vi "GageAvgSpec_orionkhw.vi"() -> ()   [LabVIEW 2016]
uses:
  <vilib>/express/express analysis/Spectral/Block/exnSpectralBlock spectral measurements power poly.vi
  <vilib>/express/express analysis/Spectral/Block/exnSpectralBlock spectral measurements power WFM.vi
  <vilib>/Utility/file.llb/Write To Spreadsheet File (DBL).vi
  <vilib>/express/express analysis/Spectral/XNode/ExpressSpectralMeasurementsBlockNode.xnode
panel:
  out "Spec(ch0)":cluster{"f0":dbl, "df":dbl, "magnitude":dbl[]}(graph)
  out "Spec(ch2)":cluster{"f0":dbl, "df":dbl, "magnitude":dbl[]}(graph)
  out "100 세트 저장완료":bool
  in  "데이터 저장 시작":bool
  out "루프 사이의 time interval":dbl
  out "Spec(ch3)":cluster{"f0":dbl, "df":dbl, "magnitude":dbl[]}(graph)
  in  "Trigger":T1={"Slope"=0, "Level"=0, "Source"=0, "External Range"=2000, "External Coupling"=0, "External"=FALSE, "Disable"=FALSE, "External Impedance"=1} {"External Impedance" items=["50 Ohm", "HiZ"]; "External Coupling" items=["DC", "AC"]; "External Range" min=2000 max=10000 step=8000; "Slope" items=["Rising", "Falling"]; "Level" min=-100 max=100; "Source" min=0 max=64 step=1}
  in  "Averages":u32=1 min=1 step=1
  in  "Averaging Method":bool
  in  "Channels":T2(array[cluster])=[{"Coupling"=0, "Differential Input"=FALSE, "Direct-to-ADC"=FALSE, "Range"=2000, "Impedance"=50, "Filter"=0}] {"Impedance" min=50 max=1000000 step=999950; "Coupling" items=["DC", "AC"]}
  in  "Acquisition":T3={"Sample Rate"=50000000.0, "Mode"=2, "Depth"=8192.0, "Segment Size"=8192.0, "Trigger Timeout"=1000000.0, "Trigger Holdoff"=0.0, "Trigger Delay"=0.0, "Clock mode"=enum."Internal"} {"Segment Size" min=256.0 step=128.0; "Trigger Holdoff" min=0.0 step=128.0; "Trigger Delay" min=0.0 step=128.0; "Depth" min=256.0 step=128.0; "Mode" items=["Single", "Dual", "Quad", "Octal"]}
  in  "Continuous":bool=TRUE
  out "Progress":string
  in  "stop":bool
  out "System Name":string
  out "Sample Bits":i32
  out "Trigger Count":i32
  out "Channel Count":i32
  out "Board Count":i32
  out "System Count":i32
  in  "Points":u32=4096
  in  "Start":i32
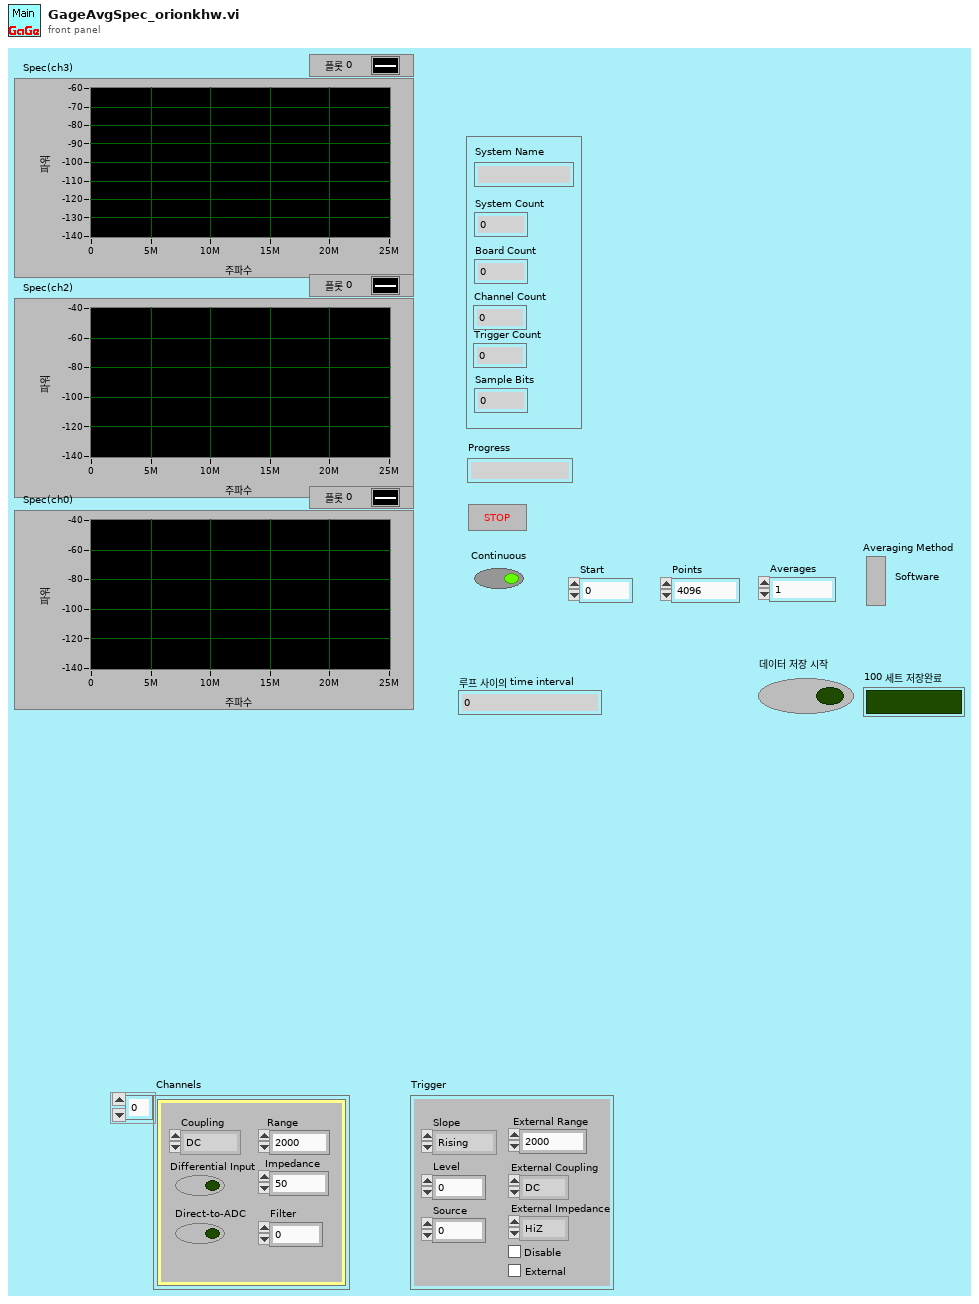
[diagram p1: front panel]
types:
  T1 = cluster{"Slope":u16, "Level":i32, "Source":i32, "External Range":u32, "External Coupling":u16, "External":bool, "Disable":bool, "External Impedance":u16}
  T2 = cluster{"Coupling":u16, "Differential Input":bool, "Direct-to-ADC":bool, "Range":u32, "Impedance":u32, "Filter":i32}[]
  T3 = cluster{"Sample Rate":dbl, "Mode":u16, "Depth":dbl, "Segment Size":dbl, "Trigger Timeout":dbl, "Trigger Holdoff":dbl, "Trigger Delay":dbl, "Clock mode":enum16{"Internal", "External", "Reference"}}
  T4 = cluster{"averaging mode":u16, "weighting mode":u16, "number of averages":u32}
  T5 = cluster{"dB On (F)":bool, "unwrap phase (F)":bool, "convert to degree (F)":bool}
  T6 = cluster{"Handle":u32, "Sample size":u32, "Resolution":i32, "Offset":i32, "Channels":u32, "Boards":u32}
  T7 = cluster{string, "Differential Input":bool, "Direct-to-ADC":bool, "Range":u32, "Impedance":u32, i32, "Filter":i32}
  T8 = cluster{"RingText.Text":string, "Level":i32, "Source":i32, "External Range":u32, "RingText.Text":string, "External":bool, "Disable":bool, "RingText.Text":string}
  T9 = cluster{"RingText.Text":string, "Level":i32, "Source":i32, "External Range":u32, "RingText.Text":string, "External":bool, "Disable":bool, "RingText.Text":string}[]
  T10 = cluster{"Handle":u32, "Sample Size":u32, "Resolution":i32, "Offset":i32, "Channels":u32, "Boards":u32}
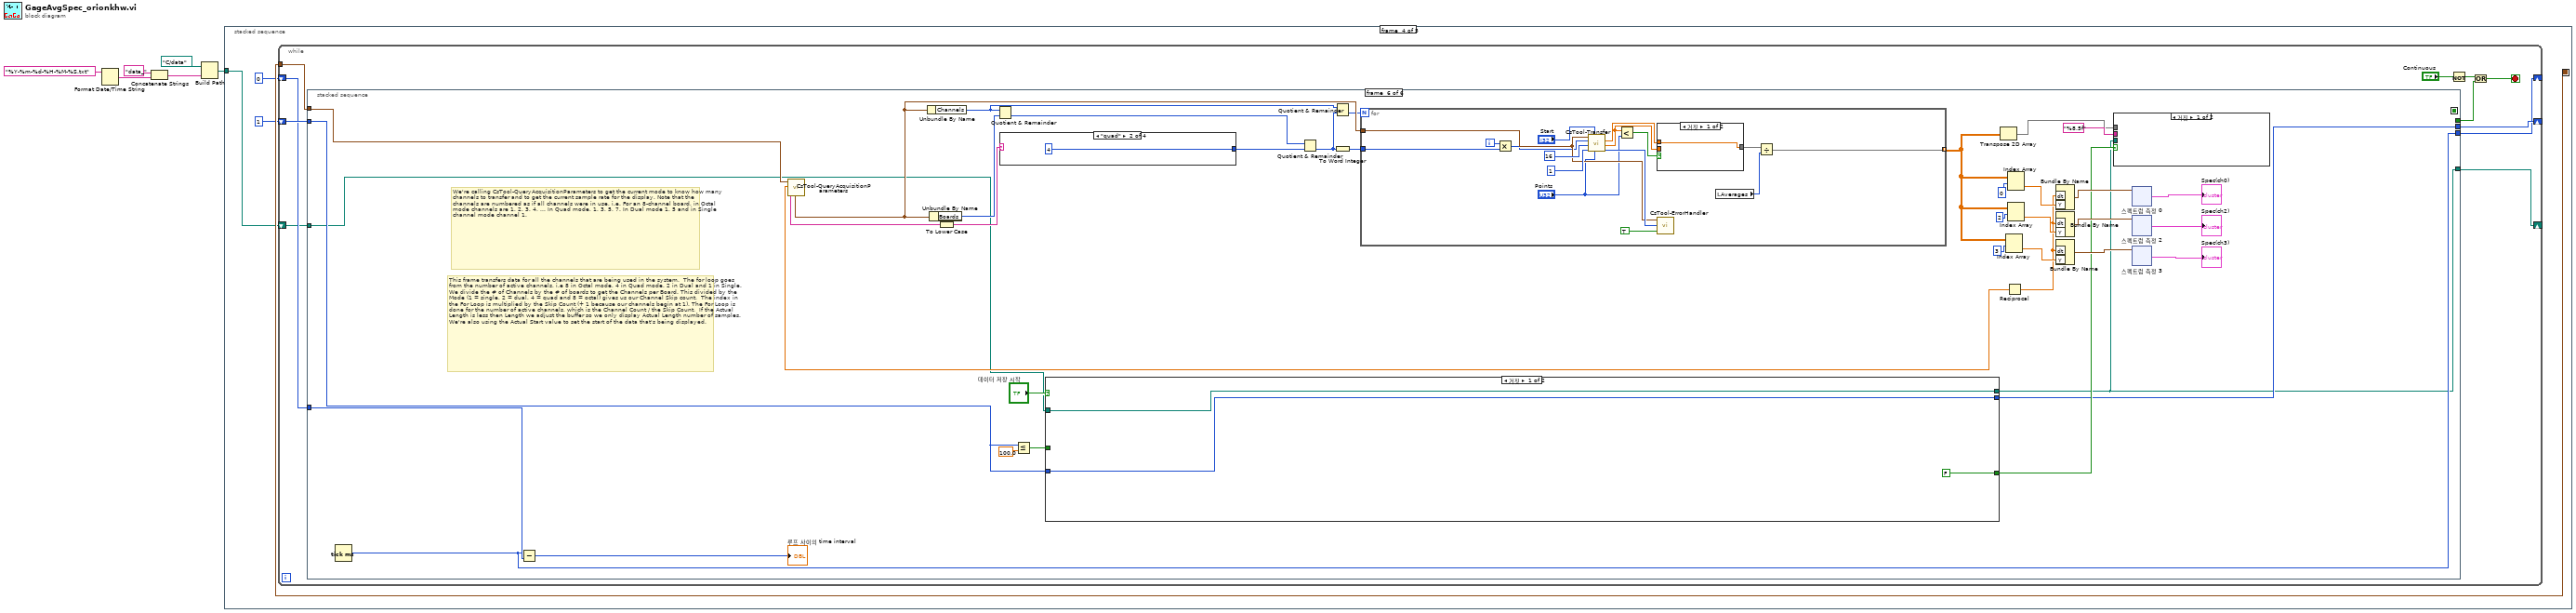
[diagram p0: block diagram]
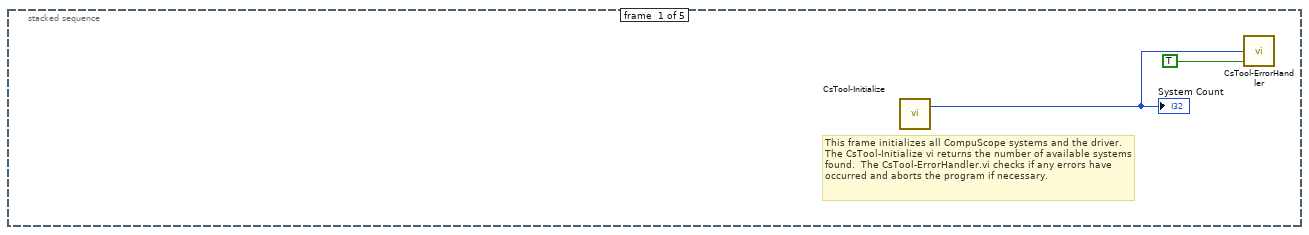
[diagram p2: hidden frame]
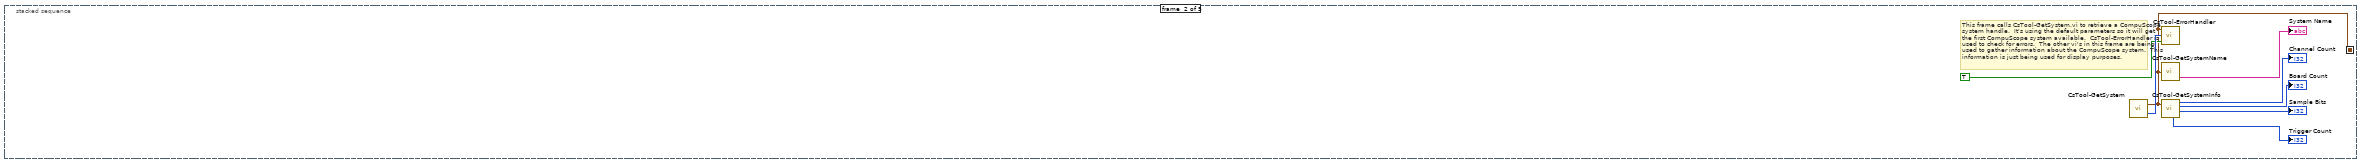
[diagram p3: hidden frame]
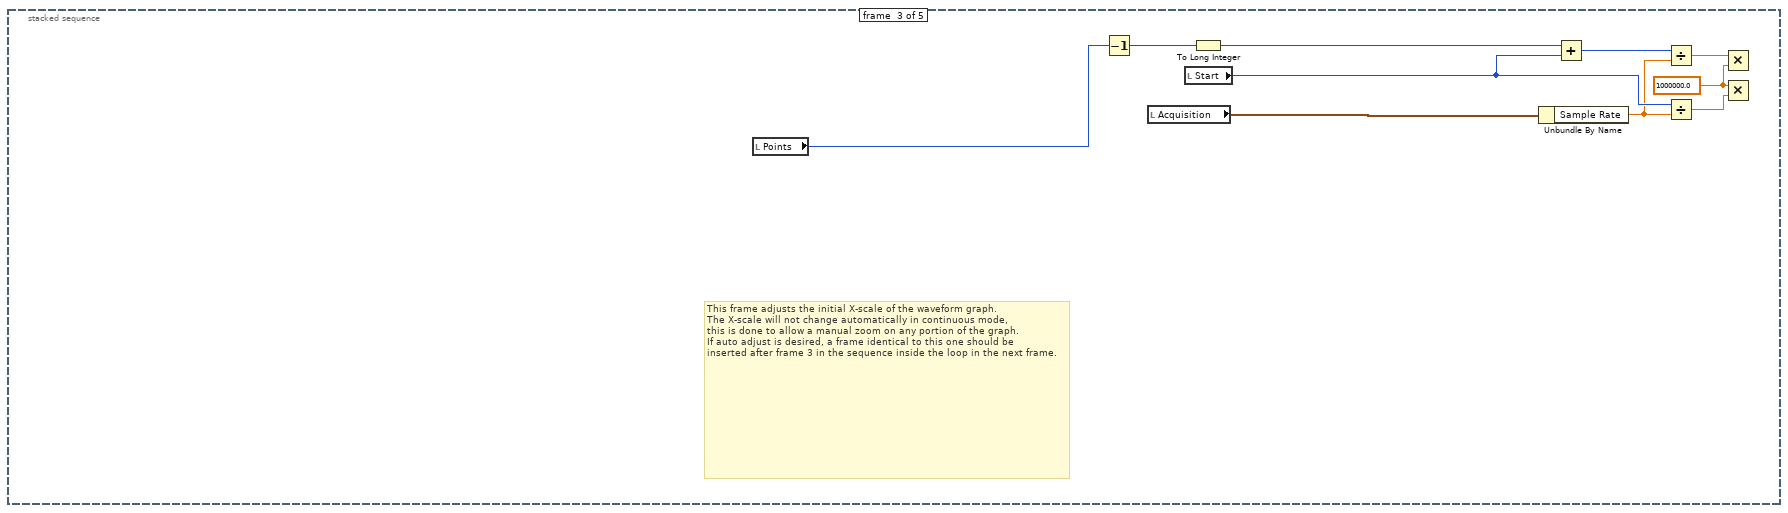
[diagram p4: hidden frame]
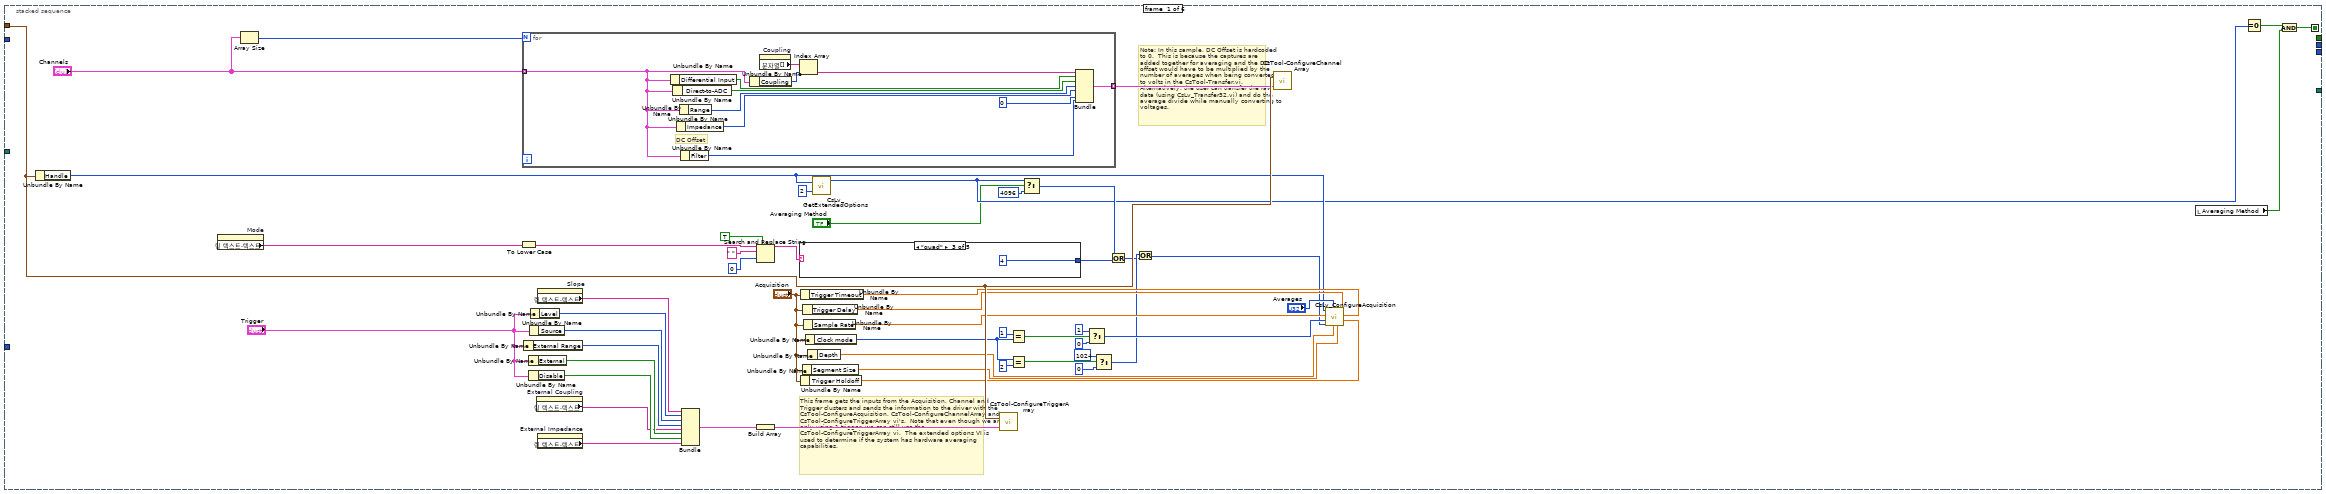
[diagram p5: hidden frame]
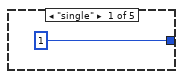
[diagram p6: hidden frame]
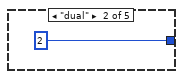
[diagram p7: hidden frame]
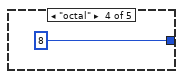
[diagram p8: hidden frame]
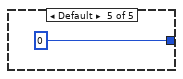
[diagram p9: hidden frame]
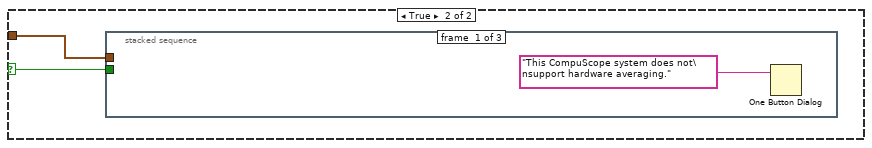
[diagram p11: hidden frame]
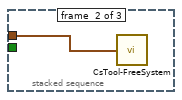
[diagram p12: hidden frame]
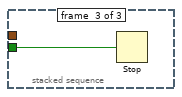
[diagram p13: hidden frame]
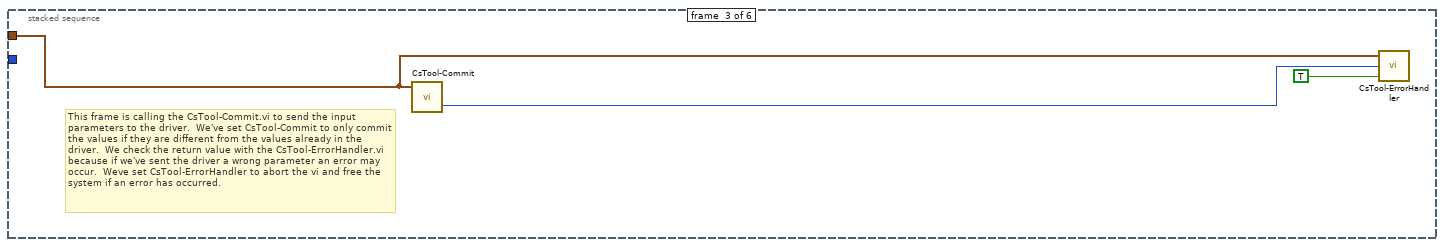
[diagram p14: hidden frame]
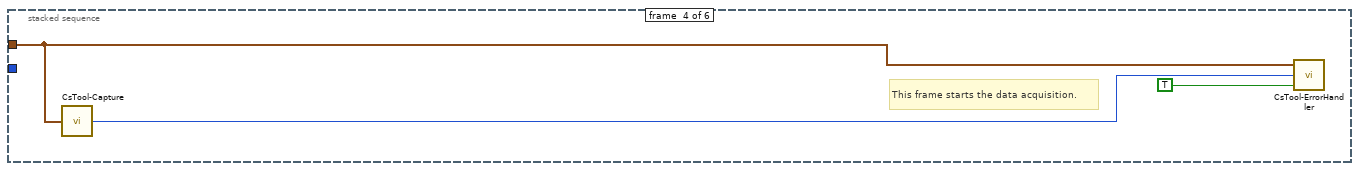
[diagram p15: hidden frame]
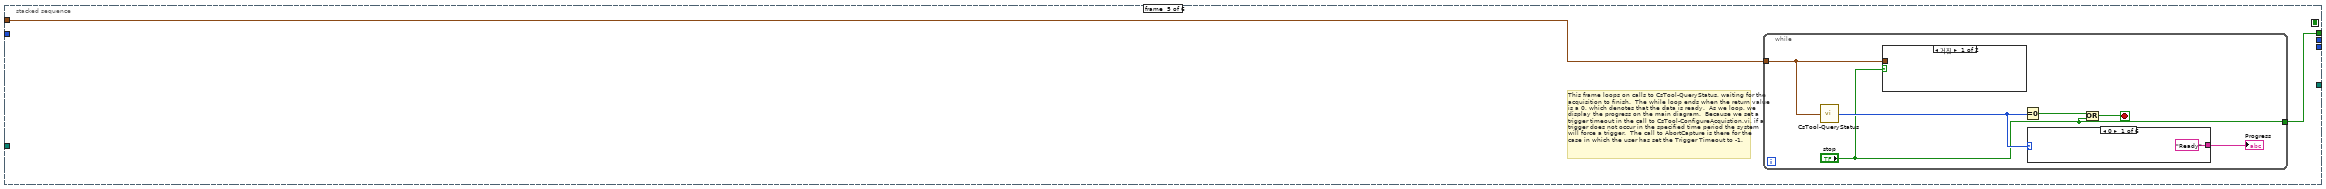
[diagram p16: hidden frame]
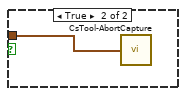
[diagram p17: hidden frame]
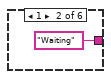
[diagram p18: hidden frame]
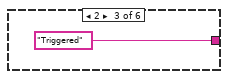
[diagram p19: hidden frame]
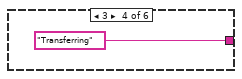
[diagram p20: hidden frame]
diagram:
  n1 = Format Date/Time String(time format string (%c)="%Y-%m-%d-%H-%M-%S.txt" ("시간 포맷 문자열 (%c)")) -> (date/time string=w2:string)  [unwired: 2 in]
  n2 = Concatenate Strings "Concatenate Strings"("data_", w2) -> (w1:string)
  n3 = Build Path(base path=path "C:/data", name or relative path=w1) -> (appended path=w4:path)
  n4 = stacked-sequence {
    seq-local: [_ w11 _ _ _] -> [_ _ _ w30 w252]
    tunnel: w4 -> [_ _ _ w27 _]
    frame #0 {
      # "This frame initializes all CompuScope systems and the driver.\nThe CsTool-Initialize vi returns the number of available systems found.  The CsTool-ErrorHandler.vi checks if any errors have occurred and aborts the program if necessary."
      n5 = call <userlib>:"CsTool-Initialize.vi"() -> ("Number Of Systems"=w8:i32)  [unwired: 1 out]
      "System Count" <- w8
      n6 = call <userlib>:"CsTool-ErrorHandler.vi"("StopOnError (true)"=TRUE, "Error Code"=w8) -> ()  [unwired: 1 in, 1 out]
    }
    frame #1 {
      # "This frame calls CsTool-GetSystem.vi to retrieve a CompuScope system handle.  It's using the default parameters so it will get the first CompuScope system available.  CsTool-ErrorHandler is used to check for errors.  The other vi's in this frame are being used to gather information about the CompuScope system.  This information is just being used for display purposes."
      n7 = call <userlib>:"CsTool-GetSystem.vi"() -> ("Error Code"=w13:i32, "Handle Cluster"=w11:T6)  [unwired: 4 in]
      n8 = call <userlib>:"CsTool-ErrorHandler.vi"("StopOnError (true)"=TRUE, "Error Code"=w13, "Handle Cluster"=w11) -> ()  [unwired: 1 out]
      n9 = call <userlib>:"CsTool-GetSystemName.vi"("Handle Cluster"=w11) -> ("System Name"=→"System Name":string)  [unwired: 1 out]
      n10 = call <userlib>:"CsTool-GetSystemInfo.vi"("Handle Cluster"=w11) -> ("Number Of Triggers"=→"Trigger Count":u32, "Number Of Channels"=→"Channel Count":u32, "Number Of Boards"=→"Board Count":u32, "Sample Bits"=→"Sample Bits":u32)  [unwired: 3 out]
    }
    frame #2 {
      w26 = 1000000.0
      # "This frame adjusts the initial X-scale of the waveform graph.\nThe X-scale will not change automatically in continuous mode, \nthis is done to allow a manual zoom on any portion of the graph.\nIf auto adjust is desired, a frame identical to this one should be\ninserted after frame 3 in the sequence inside the loop in the next frame."
      n11 = local read "Points"() -> (w23:u32)
      n12 = Decrement(x=w23) -> (x-1=w17:u32)
      n13 = local read "Acquisition"() -> (w21:T3)
      n14 = local read "Start"() -> (w24:i32)
      n15 = To Long Integer(number=w17) -> (32bit integer=w18:i32)
      n16 = Unbundle By Name(w21) -> ("Sample Rate"=w22:dbl)
      n17 = Add(x=w18, y=w24) -> (x+y=w20:i32)
      n18 = Divide(x=w20, y=w22) -> (x/y=w19:dbl)
      n19 = Divide(x=w24, y=w22) -> (x/y=w25:dbl)
      n20 = Multiply(x=w19, y=w26) -> ()  [unwired: 1 out]
      n21 = Multiply(x=w26, y=w25) -> ()  [unwired: 1 out]
    }
    frame #3 {
      n22 = while {
        tunnel: w30 -> [w41]
        shift-right: [w35] -> _
        shift-left: 1 -> [w36]
        shift-right: [w33] -> _
        shift-left: 0 -> [w34]
        shift-right: [w32] -> _
        shift-left: w27 -> [w31]
        stop <- w38 stop-if-true
        n23 = stacked-sequence {
          seq-local: [w62 _ _ _ _ _] -> [_ w111 _ _ _ _]
          tunnel: w41 -> [w87 w110 w117 w120 w124 w176]
          tunnel: [_ _ _ _ w123 _] -> w37
          tunnel: w36 -> [_ _ _ _ _ w143]
          tunnel: [_ _ _ _ _ w144] -> w35
          tunnel: w34 -> [_ _ _ _ _ w150]
          tunnel: [_ _ _ _ _ w148] -> w33
          tunnel: [_ _ _ _ _ w142] -> w32
          tunnel: w31 -> [_ _ _ _ _ w141]
          frame #0 {
            # "Note: In this sample, DC Offset is hardcoded to 0.  This is because the captures are added together for averaging and the DC offset would have to be multiplied by the number of averages when being converted to volts in the CsTool-Transfer.vi. Alternatively, the user can transfer the raw data (using CsLv_Transfer32.vi) and do the average divide while manually converting to voltages."
            # "This frame gets the inputs from the Acquisition, Channel and Trigger clusters and sends the information to the driver with the CsTool-ConfigureAcquisition, CsTool-ConfigureChannelArray and CsTool-ConfigureTriggerArray vi's.  Note that even though we are only using 1 trigger, we can still use the CsTool-ConfigureTriggerArray vi.  The extended options VI is used to determine if the system has hardware averaging capabilities."
            n24 = Unbundle By Name(w87) -> ("Handle"=w66:u32)
            n25 = property on="Mode" class="Ring (엄격한)"() -> ("링 텍스트.텍스트"=w76:string)  [unwired: 2 in, 2 out]
            n26 = Array Size(array="Channels") -> (size(s)=w88:i32)
            n27 = To Lower Case(string=w76) -> (all lower case string=w82:string)
            n28 = for {
              N: w88 -> [_]
              tunnel: "Channels" -> [w101] mode=indexing
              tunnel: [w105] -> w46 mode=indexing
              # "DC Offset"
              n29 = Unbundle By Name(w101) -> ("Differential Input"=w109:bool)
              n30 = Unbundle By Name(w101) -> ("Direct-to-ADC"=w108:bool)
              n31 = Unbundle By Name(w101) -> ("Impedance"=w106:u32)
              n32 = Unbundle By Name(w101) -> ("Range"=w107:u32)
              n33 = Unbundle By Name(w101) -> ("Filter"=w100:i32)
              n34 = Unbundle By Name(w101) -> ("Coupling"=w103:u16)
              n35 = property on="Coupling" class="Ring (엄격한)"() -> ("문자열[]"=w104:string[])  [unwired: 2 in, 2 out]
              n36 = Index Array(array=w104, index=w103) -> (element=w102:string)
              n37 = Bundle(w102, "Differential Input"=w109, "Direct-to-ADC"=w108, "Range"=w107, "Impedance"=w106, 0, "Filter"=w100) -> (w105:T7)  [unwired: 1 in]
            }
            n38 = Unbundle By Name("Trigger") -> ("External Range"=w92:u32)
            n39 = Unbundle By Name("Trigger") -> ("External"=w48:bool)
            n40 = Unbundle By Name("Trigger") -> ("Disable"=w47:bool)
            n41 = Unbundle By Name("Trigger") -> ("Source"=w49:i32)
            n42 = Unbundle By Name("Trigger") -> ("Level"=w93:i32)
            n43 = property on="External Coupling" class="Ring (엄격한)"() -> ("링 텍스트.텍스트"=w43:string)  [unwired: 2 in, 2 out]
            n44 = property on="Slope" class="Ring (엄격한)"() -> ("링 텍스트.텍스트"=w44:string)  [unwired: 2 in, 2 out]
            n45 = property on="External Impedance" class="Ring (엄격한)"() -> ("링 텍스트.텍스트"=w42:string)  [unwired: 2 in, 2 out]
            n46 = Bundle("RingText.Text"=w44, "Level"=w93, "Source"=w49, "External Range"=w92, "RingText.Text"=w43, "External"=w48, "Disable"=w47, "RingText.Text"=w42) -> (w91:T8)  [unwired: 1 in]
            n47 = Search and Replace String(replace all?=TRUE, input string=w82, search string=" ", offset=0) -> (result string=w79:string)  [unwired: 4 in, 3 out]
            n48 = Build Array(w91) -> (w90:T9)
            n49 = case shown="\"quad\"" w79 {
              tunnel: [1 2 4 8 0] -> w67
              frame "single" {
              }
              frame "dual" {
              }
              frame "quad" {
              }
              frame "octal" {
              }
              frame Default {
              }
            }
            n50 = Unbundle By Name("Acquisition") -> ("Trigger Timeout"=w73:dbl)
            n51 = Unbundle By Name("Acquisition") -> ("Trigger Holdoff"=w72:dbl)
            n52 = Unbundle By Name("Acquisition") -> ("Segment Size"=w75:dbl)
            n53 = Unbundle By Name("Acquisition") -> ("Trigger Delay"=w74:dbl)
            n54 = Unbundle By Name("Acquisition") -> ("Sample Rate"=w86:dbl)
            n55 = Unbundle By Name("Acquisition") -> ("Clock mode"=w57:enum16{"Internal", "External", "Reference"})
            n56 = Unbundle By Name("Acquisition") -> ("Depth"=w78:dbl)
            n57 = call <userlib>:"CsLv_GetExtendedOptions.vi"("Handle"=w66, "Option"=2) -> ("User Mode"=w64:u32)  [unwired: 2 out]
            n58 = call <userlib>:"CsTool-ConfigureTriggerArray.vi"("Triggers"=w90, "Handle Cluster"=w87) -> ()  [unwired: 1 out]
            n59 = Equal?(x=1, y=w57) -> (x = y?=w58:bool)
            n60 = Equal?(x=w57, y=2) -> (x = y?=w55:bool)
            n61 = Select(t=w64, s="Averaging Method", f=4096) -> (s? t:f=w68:u32)
            n62 = Select(t=u32 1, s=w58, f=u32 0) -> (s? t:f=w83:u32)
            n63 = Select(t=1024, s=w55, f=0) -> (s? t:f=w54:i32)
            n64 = Or(x=w68, y=w67) -> (x .or. y?=w52:u32)
            n65 = Or(x=w54, y=w52) -> (x .or. y?=w53:u32)
            n66 = call <userlib>:"CsTool-ConfigureChannelArray.vi"("Channels"=w46, "Handle Cluster"=w87) -> ()  [unwired: 1 out]
            n67 = call <userlib>:"CsLv_ConfigureAcquisition.vi"("Trigger Holdoff (0)"=w72, "Trigger Timeout (10000000)"=w73, "Trigger Delay (0)"=w74, "Segment Size (8192)"=w75, "Depth (8192)"=w78, "Segment Count (1)"="Averages", "Mode (2)"=w53, "External Clock (0)"=w83, "Sample Rate (100000000)"=w86, "Handle"=w66) -> ()  [unwired: 1 in, 1 out]
            n68 = local read "Averaging Method"() -> (w51:bool)
            n69 = Equal To 0?(x=w64) -> (x = 0?=w63:bool)
            n70 = And(x=w63, y=w51) -> (x .and. y?=w62:bool)
          }
          frame #1 {
            # "If, in the previous frame, the CsLv_GetExtendedOptions vi returned a 0, this means that hardware averaging is not available for this system. So if hardware averaging was chosend and the system does not support it, we will report the error, free the CompuScope system and stop the application."
            n71 = case shown="거짓" w111 {
              selector: w111 -> [_ w112]
              tunnel: w110 -> [_ w113]
              frame False {
              }
              frame True {
                n72 = stacked-sequence {
                  tunnel: w113 -> [_ w115 _]
                  tunnel: w112 -> [_ _ w116]
                  frame #0 {
                    n73 = One Button Dialog(message="This CompuScope system does not\nsupport hardware averaging.") -> ()  [unwired: 1 in, 1 out]
                  }
                  frame #1 {
                    n74 = call <userlib>:"CsTool-FreeSystem.vi"("Handle Cluster"=w115) -> ()  [unwired: 1 out]
                  }
                  frame #2 {
                    n75 = Stop(stop? (T)=w116) -> ()
                  }
                }
              }
            }
          }
          frame #2 {
            # "This frame is calling the CsTool-Commit.vi to send the input parameters to the driver.  We've set CsTool-Commit to only commit the values if they are different from the values already in the driver.  We check the return value with the CsTool-ErrorHandler.vi because if we've sent the driver a wrong parameter an error may occur.  Weve set CsTool-ErrorHandler to abort the vi and free the system if an error has occurred."
            n76 = call <userlib>:"CsTool-Commit.vi"("Handle Cluster"=w117) -> ("Error Code"=w119:i32)  [unwired: 2 in, 1 out]
            n77 = call <userlib>:"CsTool-ErrorHandler.vi"("StopOnError (true)"=TRUE, "Error Code"=w119, "Handle Cluster"=w117) -> ()  [unwired: 1 out]
          }
          frame #3 {
            # "This frame starts the data acquisition."
            n78 = call <userlib>:"CsTool-Capture.vi"("Handle Cluster"=w120) -> ("Error Code"=w122:i32)
            n79 = call <userlib>:"CsTool-ErrorHandler.vi"("StopOnError (true)"=TRUE, "Error Code"=w122, "Handle Cluster"=w120) -> ()  [unwired: 1 out]
          }
          frame #4 {
            # "This frame loops on calls to CsTool-QueryStatus, waiting for the acquisition to finish.  The while loop ends when the return value is a 0, which denotes that the data is ready.  As we loop, we display the progress on the main diagram.  Because we set a trigger timeout in the call to CsTool-ConfigureAcquistion.vi, if a trigger does not occur in the specified time period the system will force a trigger.  The call to AbortCapture is there for the case in which the user has set the Trigger Timeout to -1."
            n80 = while {
              tunnel: w124 -> [w125]
              tunnel: ["stop"] -> w123
              stop <- w127 stop-if-true
              n81 = call <userlib>:"CsTool-QueryStatus.vi"("Handle Cluster"=w125) -> ("Status"=w130:i32)
              n82 = case shown="거짓" "stop" {
                tunnel: w125 -> [_ w131]
                frame False {
                }
                frame True {
                  n83 = call <userlib>:"CsTool-AbortCapture.vi"("Handle Cluster"=w131) -> ()  [unwired: 1 out]
                }
              }
              n84 = Equal To 0?(x=w130) -> (x = 0?=w128:bool)
              n85 = case shown="0" w130 {
                tunnel: ["Ready" "Waiting" "Triggered" "Transferring" "Calibrating" " "] -> w129
                frame 0 {
                }
                frame 1 {
                }
                frame 2 {
                }
                frame 3 {
                }
                frame 4 {
                }
                frame 5, Default {
                }
              }
              "Progress" <- w129
              n86 = Or(x=w128, y="stop") -> (x .or. y?=w127:bool)
            }
          }
          frame #5 {
            # "We're calling CsTool-QueryAcquisitionParameters to get the current mode to know how many channels to transfer and to get the current sample rate for the display. Note that the channels are numbered as if all channels were in use, i.e. For an 8-channel board, in Octal mode channels are 1, 2, 3, 4, ... In Quad mode, 1, 3, 5, 7. In Dual mode 1, 5 and in Single channel mode channel 1."
            # "This frame transfers data for all the channels that are being used in the system.  The for loop goes from the number of active channels, i.e 8 in Octal mode, 4 in Quad mode, 2 in Dual and 1 in Single.  We divide the # of Channels by the # of boards to get the Channels per Board. This divided by the Mode (1 = single, 2 = dual, 4 = quad and 8 = octal) gives us our Channel Skip count.  The index in the For Loop is multiplied by the Skip Count (+ 1 because our channels begin at 1). The For Loop is done for the number of active channels, which is the Channel Count / the Skip Count.  If the Actual Length is less then Length we adjust the buffer so we only display Actual Length number of samples.  We're also using the Actual Start value to set the start of the data that's being displayed."
            n87 = Tick Count (ms)() -> (millisecond timer value=w148:u32)
            n88 = Subtract(x=w148, y=w150) -> (x-y=→"루프 사이의 time interval":u32)
            n89 = call <userlib>:"CsTool-QueryAcquisitionParameters.vi"("Handle Cluster"=w176) -> ("Output Handle Cluster"=w175:T10, "Mode"=w173:string, "Sample Rate"=w165:dbl)  [unwired: 8 out]
            n90 = Unbundle By Name(w175) -> ("Channels"=w168:u32)
            n91 = Unbundle By Name(w175) -> ("Boards"=w171:u32)
            n92 = To Lower Case(string=w173) -> (all lower case string=w172:string)
            n93 = Quotient & Remainder(x=w168, y=w171) -> (floor(x/y)=w170:u32)  [unwired: 1 out]
            n94 = case shown="\"quad\"" w172 {
              tunnel: [2 4 8 1] -> w169
              frame "dual", Default {
              }
              frame "quad" {
              }
              frame "octal" {
              }
              frame "single" {
              }
            }
            n95 = Less Or Equal?(x=w143, y=100.0) -> (x <= y?=w146:bool)
            n96 = case shown="거짓" "데이터 저장 시작" {
              tunnel: [FALSE w185] -> w145
              tunnel: w146 -> [_ w185]
              tunnel: [w179 w182] -> w144
              tunnel: w143 -> [w179 w186]
              tunnel: w141 -> [w177 w181]
              tunnel: [w177 w180] -> w142
              frame False {
              }
              frame True {
                n97 = Increment(x=w186) -> (x+1=w183:i32)
                n98 = Not(x=w185) -> (.not. x?=w184:bool)
                "100 세트 저장완료" <- w184
                n99 = property on="데이터 저장 시작" class="Bool (엄격한)"("Value"=w185) -> ()  [unwired: 2 in, 2 out]
                n100 = case shown="참" w184 {
                  tunnel: [w188 1] -> w182
                  tunnel: w183 -> [w188 _]
                  tunnel: w181 -> [w187 _]
                  tunnel: [w187 w189] -> w180
                  frame False {
                  }
                  frame True {
                    n101 = Format Date/Time String(time format string (%c)="%Y-%m-%d-%H-%M-%S.txt" ("시간 포맷 문자열 (%c)")) -> (date/time string=w191:string)  [unwired: 2 in]
                    n102 = Concatenate Strings("data_", w191) -> (w190:string)
                    n103 = Build Path(base path=path "C:/data", name or relative path=w190) -> (appended path=w189:path)
                  }
                }
              }
            }
            n104 = Quotient & Remainder(x=w170, y=w169) -> (floor(x/y)=w167:u32)  [unwired: 1 out]
            n105 = Quotient & Remainder(x=w168, y=w167) -> (floor(x/y)=w166:u32)  [unwired: 1 out]
            n106 = To Word Integer(number=w167) -> (16bit integer=w174:i16)
            n107 = for {
              N: w166 -> [_]
              tunnel: w175 -> [w236]
              tunnel: [w232] -> w157 mode=indexing
              tunnel: w174 -> [w237]
              i -> [w245]
              n108 = Multiply(x=w245, y=w237) -> (x*y=w235:i32)
              n109 = call <userlib>:"CsTool-Transfer.vi"("Length (4096)"="Points", "Start (0)"="Start", "Segment (1)"=1, "Mode (0)"=16, "Channel (0)"=w235, "Handle Cluster"=w236) -> ("Error Code"=w240:i32, "Actual Length"=w243:dbl, "Data in Volts"=w233:dbl[])  [unwired: 1 out]
              n110 = Less?(x=w243, y="Points") -> (x < y?=w246:bool)
              n111 = case shown="거짓" w246 {
                tunnel: w233 -> [w247 w251]
                tunnel: w243 -> [_ w249]
                tunnel: [w247 w248] -> w234
                frame False {
                }
                frame True {
                  n112 = Array Subset(array=w251, index=0, length=w249) -> (w248:dbl[])
                }
              }
              n113 = call <userlib>:"CsTool-ErrorHandler.vi"("StopOnError (true)"=TRUE, "Error Code"=w240, "Handle Cluster"=w236) -> ()  [unwired: 1 out]
              n114 = local read "Averages"() -> (w238:u32)
              n115 = Divide(x=w234, y=w238) -> (x/y=w232:dbl[])
            }
            n116 = Transpose 2D Array(2D array=w157) -> (transposed array=w152:dbl[][])
            n117 = Index Array(array=w157, index (row)=3 ("인덱스 (행)")) -> (element=w158:dbl[])  [unwired: 1 in]
            n118 = Reciprocal(x=w165) -> (1/x=w153:dbl)
            n119 = Index Array(array=w157, index (row)=0 ("인덱스 (행)")) -> (element=w162:dbl[])  [unwired: 1 in]
            n120 = Index Array(array=w157, index (row)=2 ("인덱스 (행)")) -> (element=w160:dbl[])  [unwired: 1 in]
            n121 = Bundle By Name("dt"=w153, "Y"=w162) -> (w163:waveform(dbl))  [unwired: 1 in]
            n122 = Bundle By Name("dt"=w153, "Y"=w160) -> (w161:waveform(dbl))  [unwired: 1 in]
            n123 = Bundle By Name("dt"=w153, "Y"=w158) -> (w159:waveform(dbl))  [unwired: 1 in]
            n124 = case shown="거짓" w145 {
              tunnel: w142 -> [_ w199]
              tunnel: "%8.5f" ("format (%.3f)") -> [_ w197]
              tunnel: w152 -> [_ w196]
              frame False {
              }
              frame True {
                n125 = call-poly <vilib>:"Write To Spreadsheet File.vi"("format (%.3f)"=w197, "append to file? (new file:F)"=TRUE, "2D data"=w196, "file path (dialog if empty)"=w199) -> ()  [unwired: 4 in, 1 out]
              }
            }
            n126 = xnode "스펙트럼 측정 0"("신호"=w163) -> ("파워 스펙트럼"=→"Spec(ch0)":cluster{"f0":dbl, "df":dbl, "magnitude":dbl[]})  [unwired: 1 in, 1 out]
            n127 = xnode "스펙트럼 측정 2"("신호"=w161) -> ("파워 스펙트럼"=→"Spec(ch2)":cluster{"f0":dbl, "df":dbl, "magnitude":dbl[]})  [unwired: 1 in, 1 out]
            n128 = xnode "스펙트럼 측정 3"("신호"=w159) -> ("파워 스펙트럼"=→"Spec(ch3)":cluster{"f0":dbl, "df":dbl, "magnitude":dbl[]})  [unwired: 1 in, 1 out]
          }
        }
        n129 = Not(x="Continuous") -> (.not. x?=w40:bool)
        n130 = Or(x=w40, y=w37) -> (x .or. y?=w38:bool)
      }
    }
    frame #4 {
      # "This frame frees the handle associated with the CompuScope system we've been using.  This allows the system to be used by another application."
      n131 = call <userlib>:"CsTool-FreeSystem.vi"("Handle Cluster"=w252) -> ()  [unwired: 1 out]
    }
  }
